vi "Test.vi"() -> ()   [LabVIEW 2020]
uses:
  g_ar_toolkit.image.lvlib
  CreateEmptyImageARGB.vi
  ARGB Colour.ctl
  g_ar_toolkit.common/Image Size (Integer).ctl
  g_ar_toolkit.common/g_ar_toolkit_common.lvlib
  Mapped Memory Access Image ARGB/Acquire.vi
  Mapped Memory Access Image ARGB/Mapped Memory Access Image ARGB.lvclass
  Mapped Memory Access Image ARGB/Release.vi
  Mapped Memory Access Image ARGB/GetMappedMemoryInfomation.vi
  DrawImageToPictureARGB.vi
panel:
  out "Picture":picture
  out "Array":u32[][](array[numeric])
  out "data value":u32[][](array[numeric])
  out "error IO":errorcluster
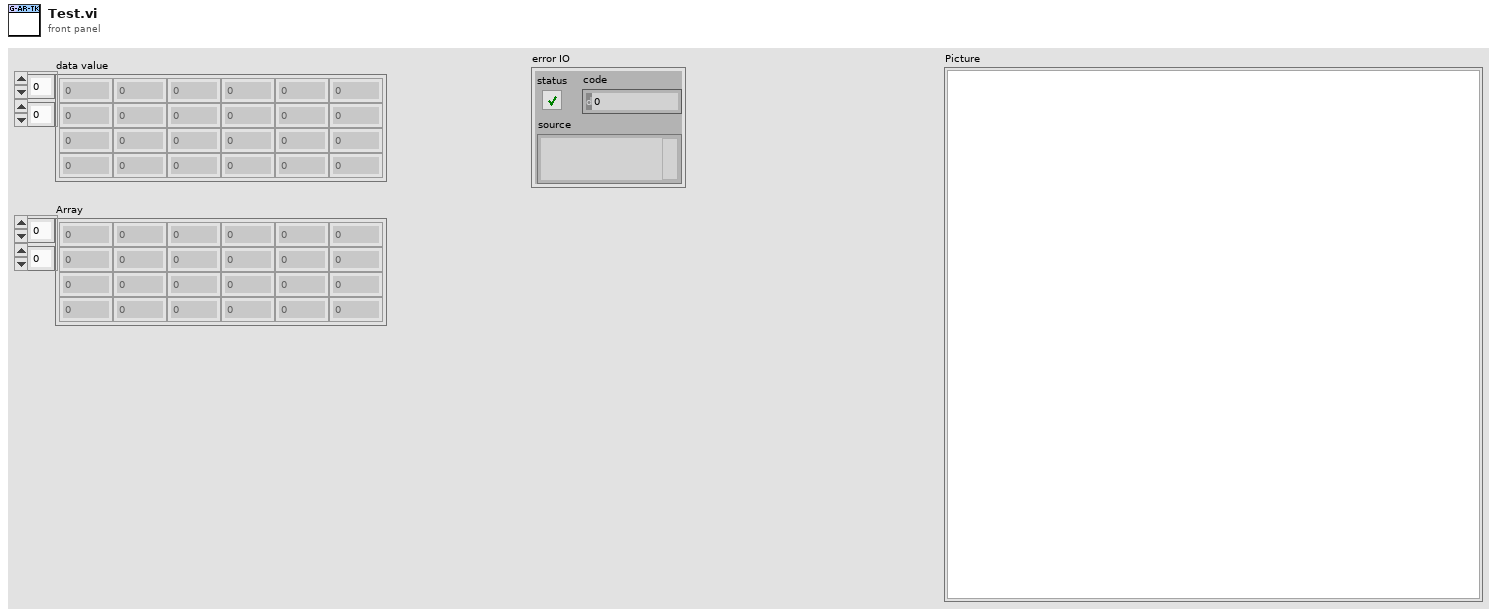
[diagram p1: front panel]
types:
  T1 = typedef "g_ar_toolkit_common.lvlib/Image Size (Integer).ctl" = cluster{"Width":u16, "Height":u16}
  T2 = typedef "g_ar_toolkit.image.lvlib/ARGB Colour.ctl" = cluster{"Alpha":u8, "RGB":u32}
  T3 = typedef "g_ar_toolkit.image.lvlib/Raw Memory Information.ctl" = cluster{"Memory Address":u64, "Dimension 0":T4, "Dimension 1":T4}
  T4 = typedef "g_ar_toolkit.image.lvlib/Raw Memory Information Dimension.ctl" = cluster{"Size":u16, "Stride":u32}
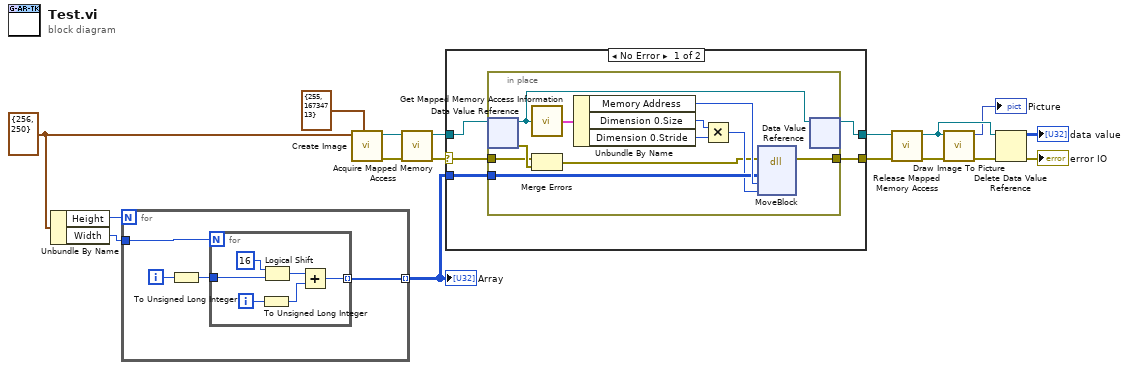
[diagram p0: block diagram]
diagram:
  w13 = T1 {"Width"=256, "Height"=250} ("Preallocated Image Size (Default: 0,0)")
  n1 = Unbundle By Name(w13) -> ("Height"=w10:u16, "Width"=w12:u16)
  n2 = for {
    N: w10 -> [_]
    tunnel: w12 -> [w21]
    tunnel: [w18] -> w11 mode=indexing
    i -> [w20]
    n3 = To Unsigned Long Integer(number=w20) -> (unsigned 32bit integer=w19:u32)
    n4 = for {
      N: w21 -> [_]
      tunnel: w19 -> [w26]
      tunnel: [w22] -> w18 mode=indexing
      i -> [w27]
      n5 = To Unsigned Long Integer(number=w27) -> (unsigned 32bit integer=w23:u32)
      n6 = Logical Shift(y=i16 16, x=w26) -> (x << y=w25:u32)
      n7 = Add(x=w25, y=w23) -> (x+y=w22:u32)
    }
  }
  "Array" <- w11
  n8 = call-poly "Create Image.vi"("Colour (Default: Black)"=T2 {"Alpha"=255, "RGB"=16734713}, "Preallocated Image Size (Default: 0,0)"=w13) -> ("error out"=w16:errorcluster, "New ARGB Image"=w8:refnum<data-value>)  [unwired: 8 in]
  n9 = call-poly "Acquire Mapped Memory Access.vi"("error in (no error)"=w16, "Image"=w8) -> ("error out"=w7:errorcluster, "Mapped Memory Access Image ARGB"=w15:refnum<data-value>)  [unwired: 8 in]
  n10 = case shown="No Error" w7 {
    selector: w7 -> [w29 w44]
    tunnel: w15 -> [w32 w45]
    tunnel: [w31 w45] -> w14
    tunnel: w11 -> [w30 _]
    tunnel: [w28 w44] -> w6
    frame No Error {
      n11 = in-place {
        in-place-border: w30 -> [w40]
        in-place-border: w29 -> [w35]
        in-place-border: [w33] -> w28
        n12 = in-place-dvr #1(w32) -> (w43:refnum<class "Mapped Memory Access Image ARGB.lvclass">, w36:errorcluster)
        n13 = call-poly "Get Mapped Memory Access Information.vi"("Mapped Memory Access Image ARGB in"=w43) -> ("Raw Memory Information"=w42:T3)
        n14 = Merge Errors(w35, w36) -> (w34:errorcluster)
        n15 = Unbundle By Name(w42) -> ("Memory Address"=w41:u64, "Dimension 0.Size"=w39:u16, "Dimension 0.Stride"=w38:u32)
        n16 = Multiply(x=w39, y=w38) -> (x*y=w37:u32)
        n17 = dll-call lib="LabVIEW" fn="MoveBlock"(error in=w34, "source"=w40, "destination"=w41, "size"=w37) -> (error out=w33:errorcluster)  [unwired: 6 in, 1 out]
        n18 = in-place-dvr #1(w43) -> (w31:refnum<data-value>)  [unwired: 1 out]
      }
    }
    frame Error {
    }
  }
  n19 = call-poly "Release Mapped Memory Access.vi"("error in (no error)"=w6, "Mapped Memory Access Image ARGB"=w14) -> ("error out"=w3:errorcluster, "Image ARGB"=w4:refnum<data-value>)  [unwired: 8 in]
  n20 = call-poly "Draw Image To Picture.vi"("error in (no error)"=w3, "ARGB Image Source"=w4) -> ("error out"=w2:errorcluster, "Picture"=→"Picture":picture)  [unwired: 8 in]
  n21 = Delete Data Value Reference(data value reference=w4, error in=w2) -> (data value=→"data value":u32[][], error out=→"error IO":errorcluster)
